vi "recordSignalLoss.vi"(8 "error in (no error)":errorcluster, 11 "Model in":refnum<class "Model.lvclass">) -> (0 "error out":errorcluster, 3 "Model out":refnum<class "Model.lvclass">)   [LabVIEW 2012, in "Model.lvclass"]
doc: "Records loss of input signal."
uses:
  Model.lvclass
  Model.lvclass/Model.ctl
  C/Program Files (x86)/National Instruments/LabVIEW 2012/user.lib/Common/ComponentModel/ComponentModel/Heartbeat/IHeartbeat/IHeartbeat.lvclass
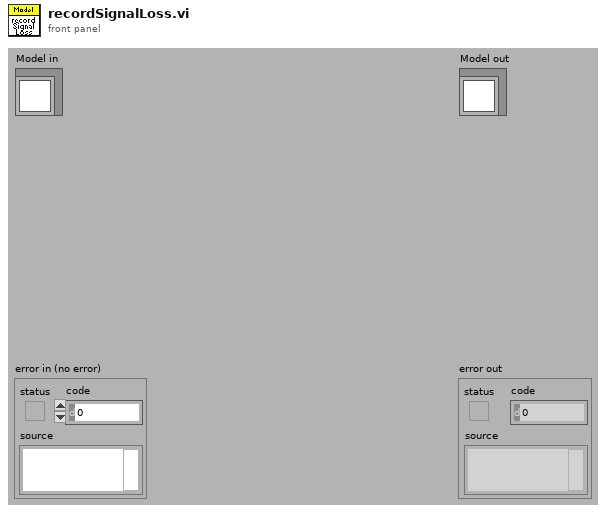
[diagram p1: front panel]
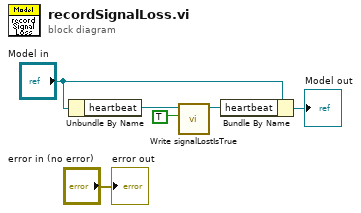
[diagram p0: block diagram]
diagram:
  n1 = Unbundle By Name("Model in") -> ("heartbeat"=w6:refnum<class "IHeartbeat.lvclass">)
  n2 = call-dynamic "Write signalLostIsTrue.vi"("signalLostIsTrue"=TRUE, "IHeartbeat in"=w6) -> ("IHeartbeat out"=w4:refnum<class "IHeartbeat.lvclass">)  [unwired: 9 in]
  n3 = Bundle By Name(cluster="Model in", "heartbeat"=w4) -> (→"Model out":refnum<class "Model.lvclass">)
  "error out" <- "error in (no error)"
